vi "manual_test_wait.vi"(7 "step_references":T1, 8 "error in (no error)":errorcluster, 11 "data":variant) -> (0 "error out":errorcluster)   [LabVIEW 2015, in "lv-recipe-machine.lvlib"]
uses:
  lv-recipe-machine.lvlib
  public/_controls/step_references.ctl
  lv-recipe-machine_/public/_controls/references.ctl
  lv-recipe-machine_/private/_controls/input.ctl
  lv-recipe-machine_/private/_controls/input_command.ctl
  lv-recipe-machine_/private/_controls/output.ctl
  lv-recipe-machine_/private/_controls/data.ctl
  lv-recipe-machine_/public/_controls/configuration.ctl
  private/_controls/recipe_data.ctl
  public/_controls/mode.ctl
  public/_controls/manual_state.ctl
  public/_controls/automatic_state.ctl
  <userlib>/antonio-alexander/lv-waitgroup/public/_controls/api_waitgroup.ctl
  public/_controls/transition.ctl
  lv-recipe-machine_/public/_controls/change.ctl
  lv-recipe-machine_/repub-dvr_nre.lvlib
  <userlib>/antonio-alexander/lv-waitgroup/lv-waitgroup.lvlib
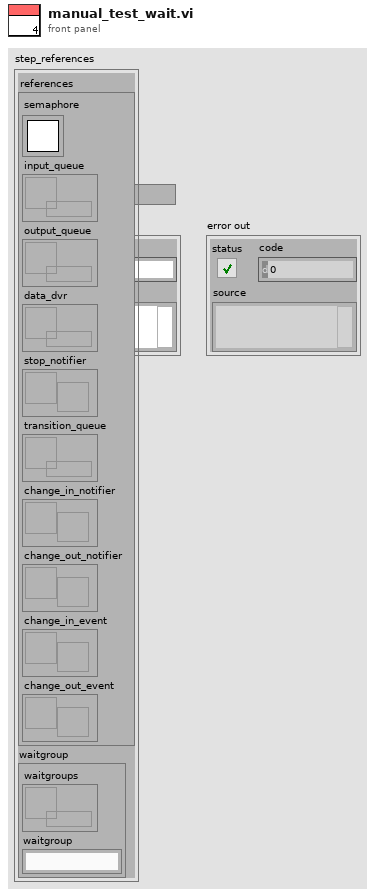
[diagram p1: front panel]
types:
  T1 = typedef "lv-recipe-machine.lvlib/step_references.ctl" = cluster{"references":T2, "api_waitgroup":T4}
  T2 = typedef "repub-dvr_nre.lvlib/references.ctl" = cluster{"semaphore":T3, "input_queue":refnum<queue>, "output_queue":refnum<queue>, "data_dvr":refnum<data-value>, "stop_notifier":refnum<notifier>, "transition_queue":refnum<queue>, "change_in_notifier":refnum<notifier>, "change_out_notifier":refnum<notifier>, "change_in_event":refnum<user-event>, "change_out_event":refnum<user-event>}
  T3 = typedef "Semaphore RefNum" = refnum<k1>
  T4 = typedef "lv-waitgroup.lvlib/api_waitgroup.ctl" = cluster{"waitgroups":refnum<data-value>, "waitgroup":string}
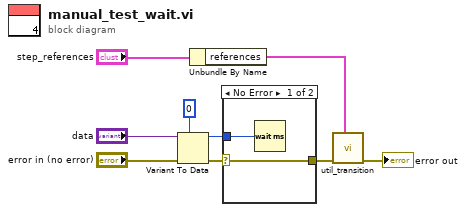
[diagram p0: block diagram]
diagram:
  n1 = Variant To Data(error in="error in (no error)", type=u32 0, Variant="data") -> (data=w5:u32, error out=w2:errorcluster)
  n2 = Unbundle By Name("step_references") -> ("references"=w9:T2)
  n3 = case shown="No Error" w2 {
    selector: w2 -> [w10 w12]
    tunnel: w5 -> [w11 _]
    tunnel: [w10 w12] -> w1
    frame No Error {
      n4 = Wait (ms)(milliseconds to wait=w11) -> ()  [unwired: 1 out]
    }
    frame Error {
    }
  }
  n5 = call "util_transition.vi"("references"=w9, "error in (no error)"=w1) -> ("error out"=→"error out":errorcluster)  [unwired: 9 in]
